vi "Read_SpillID_file.vi"(8 "error in":errorcluster, 11 "file in":path) -> (0 "error out":errorcluster, 1 "get_sid":u32, 2 "line":string="\n", 3 "file out":path)   [LabVIEW 2018, in "6509.lvlib"]
uses:
  Libraries/6509/6509.lvlib
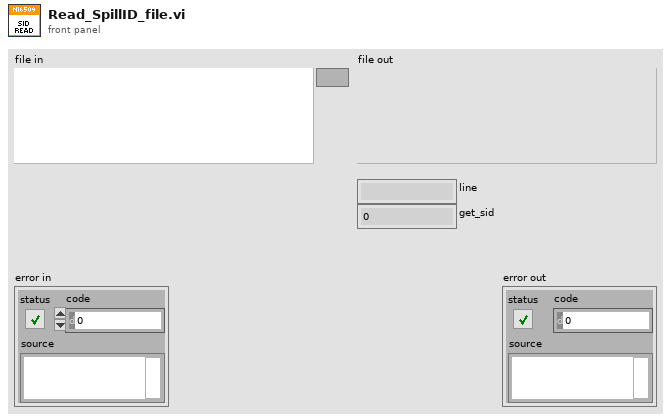
[diagram p1: front panel]
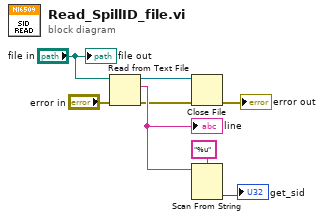
[diagram p0: block diagram]
diagram:
  n1 = Read from Text File(file (use dialog)="file in", error in="error in") -> (refnum out=w3:refnum<file>, text=w7:string, error out=w1:errorcluster)  [unwired: 2 in, 1 out]
  "line" <- w7
  n2 = Close File(refnum=w3, error in=w1) -> (error out=→"error out":errorcluster)  [unwired: 1 out]
  n3 = Scan From String(format string="%u", input string=w7) -> (output 1=→"get_sid":u32)  [unwired: 3 in, 3 out]
  "file out" <- "file in"
